vi "from_flattened_string.vi"(5 "DataString in":refnum<class "DataString.lvclass">, 8 "error in (no error)":errorcluster, 11 "string_data":string) -> (0 "error out":errorcluster, 3 "DataString out":refnum<class "DataString.lvclass">)   [LabVIEW 2020, in "variant.lvlib" / "data.lvlib" / "DataString.lvclass"]
uses:
  DataString.lvclass
  DataString.lvclass/DataString.ctl
  Bytes/Bytes.lvclass
  C:/projects/OpenG-Variant-Data-Library/source/library/Bytes/Bytes.lvclass
  C:/projects/OpenG-Variant-Data-Library/source/library/LVData/DataString/DataString.lvclass
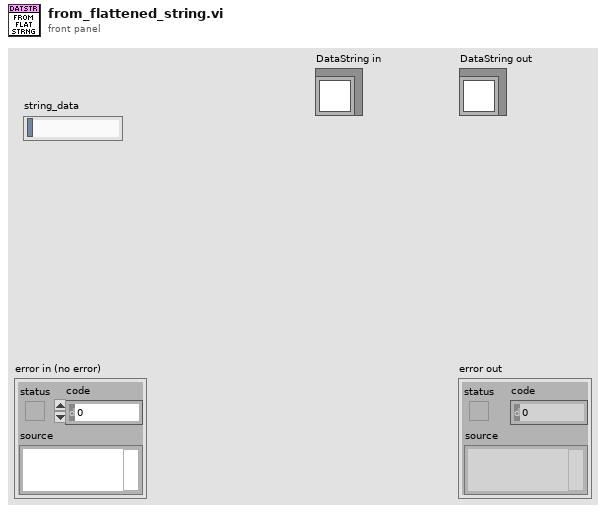
[diagram p1: front panel]
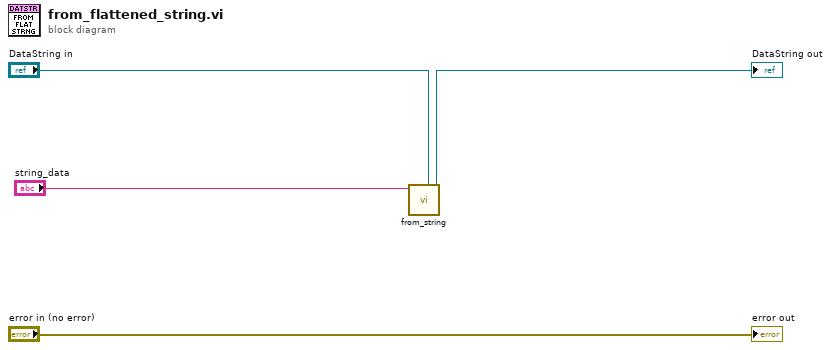
[diagram p0: block diagram]
diagram:
  n1 = call "from_string.vi"("type"="DataString in", "string_data"="string_data") -> ("Bytes out"=→"DataString out":refnum<class "DataString.lvclass">)  [unwired: 9 in]
  "error out" <- "error in (no error)"
